vi "_Parse SEM Margin List.vi"(8 "error in (no error)":errorcluster, 10 "Input String":string, 11 "VISA resource name":refnum<visa-resource-name>) -> (0 "error out":errorcluster, 1 "Results":T1(array[cluster]) {"Margin Pos Y" format="%^.3e"; "Margin Pos X" format="%^.3e"}, 2 "Reliability":i32, 3 "VISA resource name out":refnum<visa-resource-name>)   [LabVIEW 2020, in "Rohde&Schwarz CMXP NR FR2 Measurement.lvlib"]
uses:
  <instrlib>/Rohde&Schwarz CMXP NR FR2 Measurement/Rohde&Schwarz CMXP NR FR2 Measurement.lvlib
  <instrlib>/Rohde&Schwarz CMXP NR FR2 Measurement/Private/rsidr_core.llb/rsidr_core.lvlib
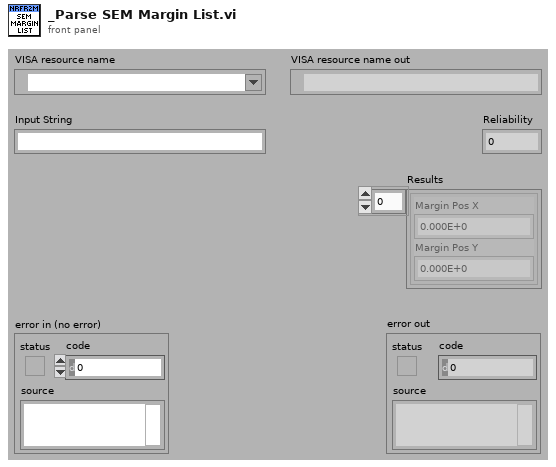
[diagram p1: front panel]
types:
  T1 = cluster{"Margin Pos X":dbl, "Margin Pos Y":dbl}[]
  T2 = cluster{"Nr Res Blocks":i32, "Offset Res Blocks":i32}
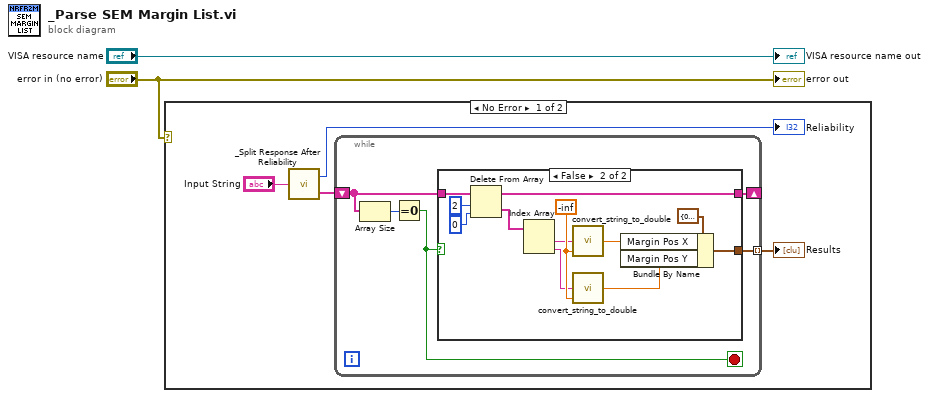
[diagram p0: block diagram]
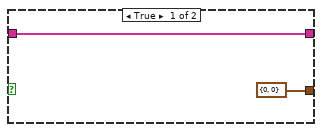
[diagram p2: hidden frame]
diagram:
  n1 = case shown="No Error" "error in (no error)" {
    frame No Error {
      n2 = call <instrlib>:"_Split Response After Reliability.vi"("Input String"="Input String") -> ("Response out"=w3:string[], "Reliability out"=→"Reliability":i32)
      n3 = while {
        tunnel: [w11] -> w4 mode=indexing
        shift-right: [w8] -> _
        shift-left: w3 -> [w10]
        stop <- w7 stop-if-true
        n4 = Array Size(array=w10) -> (size(s)=w9:i32)
        n5 = Equal To 0?(x=w9) -> (x = 0?=w7:bool)
        n6 = case shown="False" w7 {
          tunnel: [T2 {"Nr Res Blocks"=0, "Offset Res Blocks"=0} ("Detected Allocation") w24] -> w11
          tunnel: w10 -> [w12 w19]
          tunnel: [w12 w18] -> w8
          frame True {
          }
          frame False {
            w25 = -inf
            n7 = Delete From Array(array=w19, length=2, index=0) -> (deleted portion=w15:string[], array with subset deleted=w18:string[])
            n8 = Index Array(array=w15) -> (element #1=w21:string, element #2=w20:string)  [unwired: 2 in]
            n9 = call <instrlib>:"convert_string_to_double.vi"("default (0)"=w25, "String in"=w21) -> ("double value out"=w23:dbl)  [unwired: 3 in]
            n10 = call <instrlib>:"convert_string_to_double.vi"("default (0)"=w25, "String in"=w20) -> ("double value out"=w22:dbl)  [unwired: 3 in]
            n11 = Bundle By Name(cluster=cluster{"Margin Pos X":dbl, "Margin Pos Y":dbl} {"Margin Pos X"=0.0, "Margin Pos Y"=0.0} ("Margin Position"), "Margin Pos X"=w23, "Margin Pos Y"=w22) -> (w24:cluster{"Margin Pos X":dbl, "Margin Pos Y":dbl})
          }
        }
      }
      "Results" <- w4
    }
    frame Error {
    }
  }
  "VISA resource name out" <- "VISA resource name"
  "error out" <- "error in (no error)"
